vi "Sequence Read.vi"(8 "error in (no error)":errorcluster, 11 "MSX-E3701 in":refnum<class "MSX-E3701.lvclass">) -> (0 "error out":errorcluster, 1 "Control Data":T3, 2 "Acquisition Data":T1, 3 "MSX-E3701 out":refnum<class "MSX-E3701.lvclass">)   [LabVIEW 2014, in "MSX-E3701.lvlib" / "MSX-E3701.lvclass"]
doc: "Inicia la lectura de datos y los afecta a estos con la ganancia y el offset que previamente se configuraron."
uses:
  MSX-E3701.lvclass
  DriverMasterSync/build/DriverMasterSync.lvlibp/APIs/Data Queue/Control Data Cluster.ctl
  DriverMasterSync/build/DriverMasterSync.lvlibp/APIs/Data Queue/Acquisition Data Cluster.ctl
  DriverMasterSync/build/DriverMasterSync.lvlibp/APIs/Data Queue/Acquisition Data 1 Sample Cluster.ctl
  MSX-E3701.lvclass/MSX-E3701.ctl
  API/MSX-E3701_dll.lvlib
  DriverMasterSync/build/DriverMasterSync.lvlibp/Modules/HAL/DriverMasterSync/DriverMasterSyncClass/DriverMasterSync.lvclass
  DriverMasterSync/build/DriverMasterSync.lvlibp/APIs/Data Queue/WINFAS 2 Data Queue.lvlib
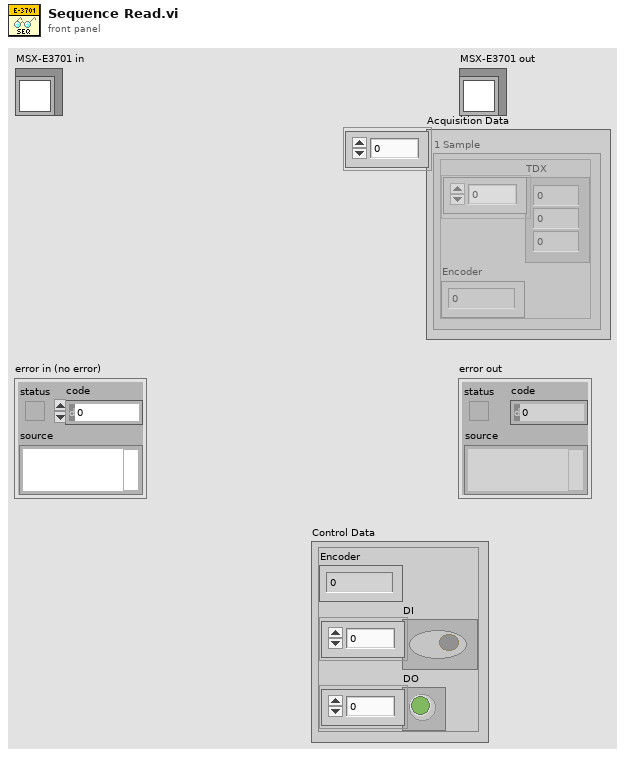
[diagram p1: front panel]
types:
  T1 = typedef "DriverMasterSync.lvlibp/WINFAS 2 Data Queue.lvlib/Acquisition Data Cluster.ctl" = T2[]
  T2 = typedef "DriverMasterSync.lvlibp/WINFAS 2 Data Queue.lvlib/Acquisition Data 1 Sample Cluster.ctl" = cluster{"TDX":sgl[], "Encoder":sgl}
  T3 = typedef "DriverMasterSync.lvlibp/WINFAS 2 Data Queue.lvlib/Control Data Cluster.ctl" = cluster{"Encoder":sgl, "DI":bool[], "DO":bool[]}
  T4 = typedef "DriverMasterSync.lvlibp/HAL Config Data.ctl" = cluster{"HWSync Index":u32, "Driver Name":string, "Channel Mask":u64}
  T5 = typedef "MSX-E3701_dll.lvlib/Connection Data.ctl" = cluster{"MX370x refnum":refnum<k24>, "IP":string, "Connection ID ":refnum<k5>, "MXCommon refnum":refnum<k24>}
  T6 = typedef "MSX-E3701_dll.lvlib/Config Data.ctl" = cluster{"Auto Refresh":cluster{"Average Mode":u64, "Average Value":u64, "Division Factor":u64, "Trigger Action":u64, "Hardware Trigger Count":u64, "Hardware Trigger Filter Time":u64, "By Trigger Nbr Of Seq To Acquire":u64, "Time stamp":bool, "Analog Output(mm)":bool, "Invert value":bool}, "Gain":sgl[], "Offset":sgl[], "Index":u64, "Range":sgl, "Sequence":cluster{"Division Factor":u64, "Nbr Of Sequence":u64, "Nbr Max Sequence To Transfer":u64, "Sequence.Delay Mode":u64, "Delay Time Unit":u64, "Delay Value":u64, "Trigger Action":u64, "Hardware Trigger Count":u64, "Hardware Trigger Filter Time":u64, "By Trigger Nbr Of Seq To Acquire":u64, "Time stamp":bool, "Sequence counter information":bool, "Analog Output(mm)":bool, "Invert value":bool, "Relative Time Stamp":bool, "Hardware trigger information":bool}, "Enable DIO":bool}
  T7 = typedef "MSX-E3701_dll.lvlib/Adquisition Data.ctl" = cluster{"Adq. Sequence":cluster{"TSs - TSu - NAS":u64[][], "Adquisition Value":u32[][], "Status IO Port":bool[]}, "Adq. Auto Refresh":cluster{"Adquisition Value":u64[], "Status IO Port":bool[], "Counter value":u64[]}}
  T8 = cluster{"TSs - TSu - NAS":u64[][], "Adquisition Value":u32[][], "Status IO Port":bool[]}
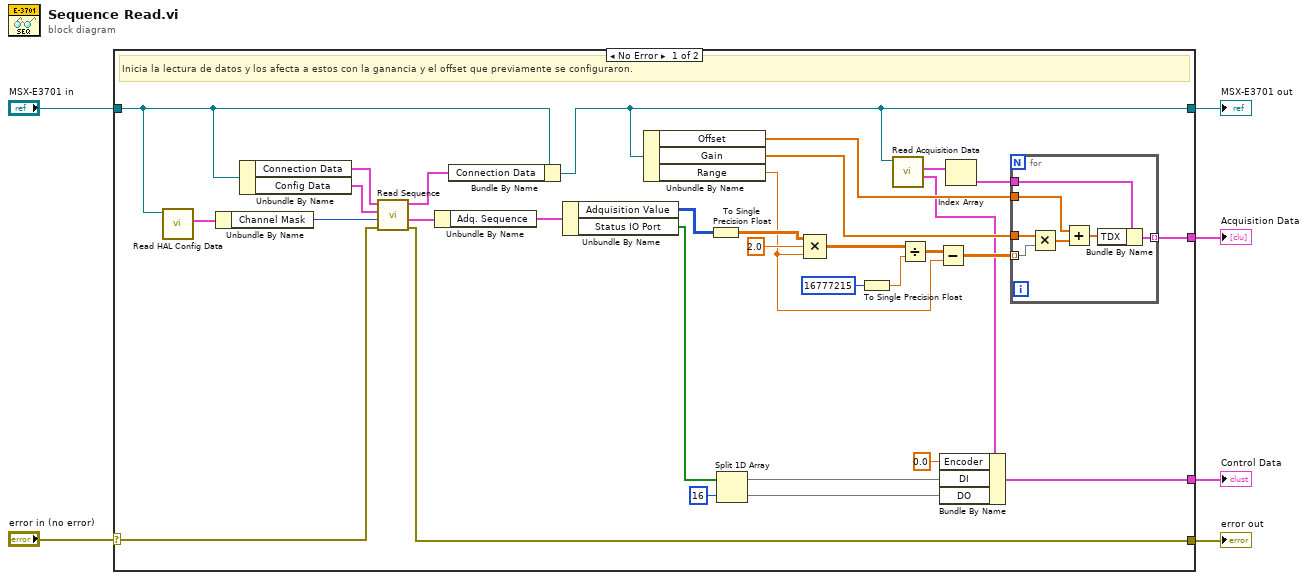
[diagram p0: block diagram]
diagram:
  n1 = case shown="No Error" "error in (no error)" {
    selector: "error in (no error)" -> [w33 w47]
    tunnel: [w9 w47] -> w5
    tunnel: [w26 w46] -> w3
    tunnel: "MSX-E3701 in" -> [w24 w46]
    tunnel: [w8 _] -> w1
    tunnel: [w27 _] -> w2
    frame No Error {
      # "Inicia la lectura de datos y los afecta a estos con la ganancia y el offset que previamente se configuraron."
      n2 = call "Read HAL Config Data.vi"("DriverMasterSync in"=w24) -> ("HAL Config Data"=w23:T4)  [unwired: 8 in, 2 out]
      n3 = Unbundle By Name(w23) -> ("Channel Mask"=w22:u64)
      n4 = Unbundle By Name(w24) -> ("Connection Data"=w35:T5, "Config Data"=w34:T6)
      n5 = call "Read Sequence.vi"("error in (no error)"=w33, "Channel Mask"=w22, "Config Data"=w34, "Connection Data In"=w35) -> ("error out"=w9:errorcluster, "Adquisition Data Out"=w31:T7, "Connection Data Out"=w32:T5)  [unwired: 5 in]
      n6 = Unbundle By Name(w31) -> ("Adq. Sequence"=w30:T8)
      n7 = Bundle By Name(cluster=w24, "Connection Data"=w32) -> (w26:refnum<class "MSX-E3701.lvclass">)
      n8 = Unbundle By Name(w30) -> ("Adquisition Value"=w15:u32[][], "Status IO Port"=w29:bool[])
      n9 = Unbundle By Name(w26) -> ("Offset"=w20:sgl[], "Gain"=w21:sgl[], "Range"=w11:sgl)
      n10 = To Single Precision Float(number=w15) -> (single precision float=w14:sgl[][])
      n11 = Split 1D Array(array=w29, index=16) -> (first subarray=w38:bool[], second subarray=w37:bool[])
      n12 = Compound Arithmetic op=MULTIPLY(w14, sgl 2.0 ("x"), w11) -> (w17:sgl[][])
      n13 = To Single Precision Float(number=u64 16777215 ("x")) -> (single precision float=w13:sgl)
      n14 = call "Read Acquisition Data.vi"("DriverMasterSync in"=w26) -> ("Control Data"=w7:T3, "Acquisition Data"=w10:T1)  [unwired: 7 in, 2 out]
      n15 = Divide(x=w17, y=w13) -> (x/y=w18:sgl[][])
      n16 = Subtract(x=w18, y=w11) -> (x-y=w16:sgl[][])
      n17 = Bundle By Name(cluster=w7, "Encoder"=sgl 0.0, "DI"=w38, "DO"=w37) -> (w27:T3)
      n18 = Index Array(array=w10) -> (element=w28:T2)  [unwired: 1 in]
      n19 = for {
        tunnel: w28 -> [w45]
        tunnel: w16 -> [w43] mode=indexing
        tunnel: w21 -> [w42]
        tunnel: w20 -> [w41]
        tunnel: [w39] -> w8 mode=indexing
        n20 = Multiply(x=w42, y=w43) -> (x*y=w44:sgl[])
        n21 = Add(x=w41, y=w44) -> (x+y=w40:sgl[])
        n22 = Bundle By Name(cluster=w45, "TDX"=w40) -> (w39:T2)
      }
    }
    frame Error {
    }
  }
  "error out" <- w5
  "MSX-E3701 out" <- w3
  "Control Data" <- w2
  "Acquisition Data" <- w1
